vi "From Value.vi"(8 "error in (no error)":errorcluster, 10 "PV Data in":refnum<class "PV Data.lvclass">, 11 "NT Scalar (Numeric) in":refnum<class "NT Scalar (Numeric).lvclass">) -> (0 "error out":errorcluster, 2 "PV Data out":refnum<class "PV Data.lvclass">, 3 "NT Scalar (Numeric) out":refnum<class "NT Scalar (Numeric).lvclass">)   [LabVIEW 2020, in "PV Access.lvlib" / "PV Data.lvlib" / "NT Scalar (Numeric).lvclass"]
uses:
  NT Scalar (Numeric).lvclass
  NT Scalar (Numeric).lvclass/NT Scalar (Numeric).ctl
  PV Data/PV Data.lvclass
  NT Scalar/NT Scalar.lvclass
  PV Data/Read Field (String).vi
  PV Data/Read Field (Variant).vi
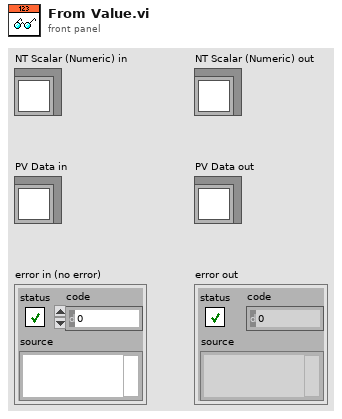
[diagram p1: front panel]
types:
  T1 = typedef "PV Access.lvlib/PV Data.lvlib/Alarm Limits.ctl" = cluster{"Active":bool, "Low Alarm Limit":variant, "Low Warning Limit":variant, "High Warning Limit":variant, "High Alarm Limit":variant, "Low Alarm Severity":T2, "Low Warning Severity":T2, "High Warning Severity ":T2, "High Alarm Severity":T2, "Hysteresis":dbl}
  T2 = typedef "PV Access.lvlib/PV Data.lvlib/Alarm Severity.ctl" = enum32{"no", "minor", "major", "record", "invalid", "undefined", ""}
  T3 = typedef "PV Access.lvlib/PV Data.lvlib/Control Metadata.ctl" = cluster{"Limit Low":variant, "Limit High":variant, "Min Step":variant}
  T4 = typedef "PV Access.lvlib/PV Data.lvlib/Display Form.ctl" = enum32{"Default", "String", "Binary", "Decimal", "Hex", "Exponential", "Engineering"}
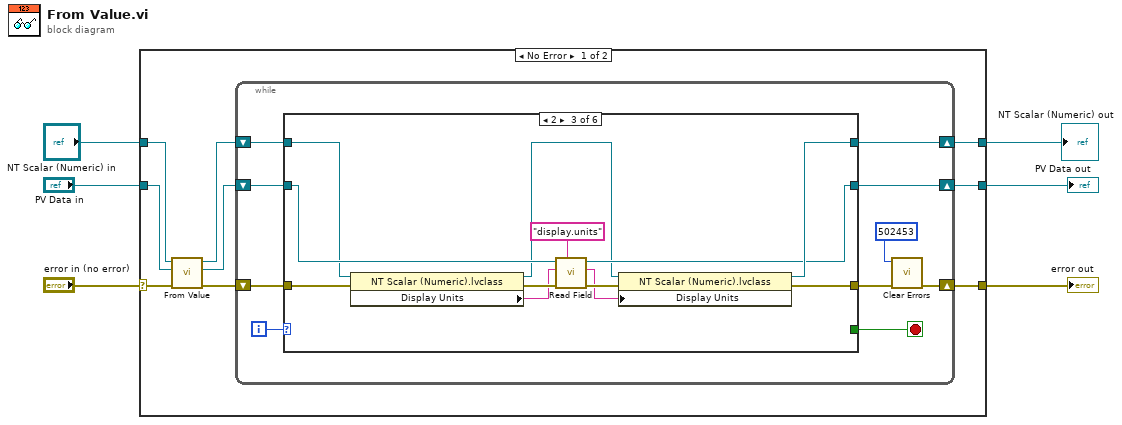
[diagram p0: block diagram]
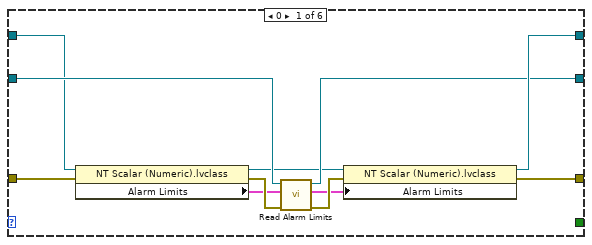
[diagram p2: hidden frame]
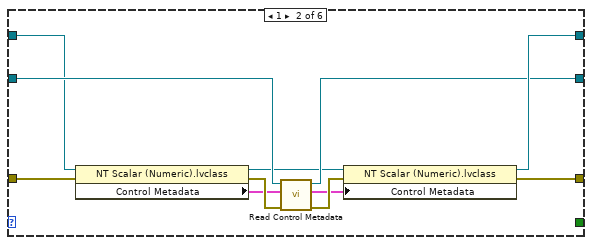
[diagram p3: hidden frame]
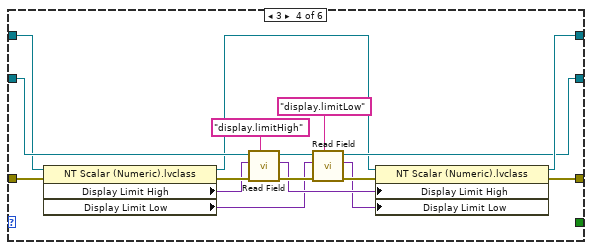
[diagram p4: hidden frame]
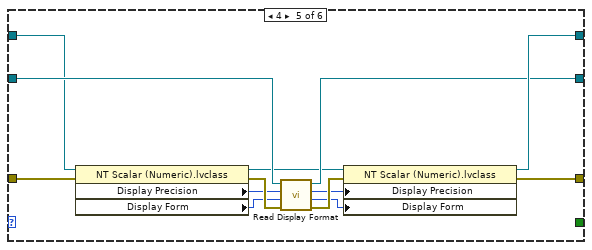
[diagram p5: hidden frame]
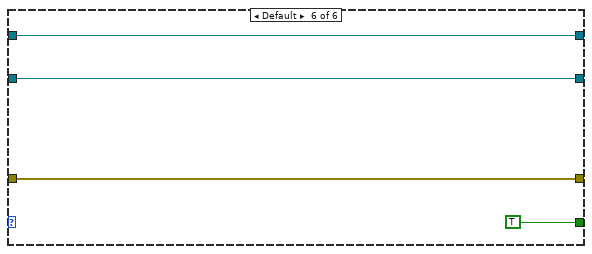
[diagram p6: hidden frame]
diagram:
  n1 = case shown="No Error" "error in (no error)" {
    selector: "error in (no error)" -> [w14 w96]
    tunnel: [w9 w96] -> w6
    tunnel: [w8 w94] -> w5
    tunnel: [w7 w95] -> w4
    tunnel: "PV Data in" -> [w13 w94]
    tunnel: "NT Scalar (Numeric) in" -> [w12 w95]
    frame No Error {
      n2 = call-parent "From Value.vi"("error in (no error)"=w14, "PV Data in"=w13, "NT Base in"=w12) -> ("error out"=w15:errorcluster, "PV Data out"=w11:refnum<class "PV Data.lvclass">, "NT Base out"=w10:refnum<class "NT Scalar (Numeric).lvclass">)  [unwired: 6 in]
      n3 = while {
        shift-right: [w21] -> w9
        shift-left: w15 -> [w23]
        shift-right: [w16] -> w8
        shift-left: w11 -> [w19]
        shift-right: [w17] -> w7
        shift-left: w10 -> [w18]
        i -> [w25]
        stop <- w24 stop-if-true
        n4 = case shown="2" w25 {
          tunnel: [_ _ _ _ _ TRUE] -> w24
          tunnel: w23 -> [w29 w40 w52 w67 w82 w92]
          tunnel: [w36 w47 w59 w76 w89 w92] -> w20
          tunnel: w19 -> [w34 w44 w53 w73 w87 w90]
          tunnel: w18 -> [w27 w38 w48 w61 w79 w91]
          tunnel: [w33 w43 w58 w75 w88 w91] -> w17
          tunnel: [w32 w42 w54 w69 w86 w90] -> w16
          frame 0 {
            n5 = property class="NT Scalar (Numeric).lvclass"(reference=w27, error in=w29) -> (reference out=w26:refnum<class "NT Scalar (Numeric).lvclass">, error out=w30:errorcluster, "Alarm Limits"=w28:T1)
            n6 = call "Read Alarm Limits.vi"("error in"=w30, "alarm limits in"=w28, "PV Data in"=w34) -> ("error out"=w35:errorcluster, "alarm limits out"=w31:T1, "PV Data out"=w32:refnum<class "PV Data.lvclass">)  [unwired: 5 in, 1 out]
            n7 = property class="NT Scalar (Numeric).lvclass"(reference=w26, error in=w35, "Alarm Limits"=w31) -> (reference out=w33:refnum<class "NT Scalar (Numeric).lvclass">, error out=w36:errorcluster)
          }
          frame 1 {
            n8 = property class="NT Scalar (Numeric).lvclass"(reference=w38, error in=w40) -> (reference out=w39:refnum<class "NT Scalar (Numeric).lvclass">, error out=w41:errorcluster, "Control Metadata"=w37:T3)
            n9 = call "Read Control Metadata.vi"("error in"=w41, "control metadata in"=w37, "PV Data in"=w44) -> ("error out"=w46:errorcluster, "control metadata out"=w45:T3, "PV Data out"=w42:refnum<class "PV Data.lvclass">)  [unwired: 5 in, 1 out]
            n10 = property class="NT Scalar (Numeric).lvclass"(reference=w39, error in=w46, "Control Metadata"=w45) -> (reference out=w43:refnum<class "NT Scalar (Numeric).lvclass">, error out=w47:errorcluster)
          }
          frame 2 {
            n11 = property class="NT Scalar (Numeric).lvclass"(reference=w48, error in=w52) -> (reference out=w49:refnum<class "NT Scalar (Numeric).lvclass">, error out=w51:errorcluster, "Display Units"=w50:string)
            n12 = call-poly "Read Field.vi"("field name"="display.units", "error in (no error)"=w51, "default"=w50, "PV Data in"=w53) -> ("error out"=w56:errorcluster, "value"=w55:string, "PV Data out"=w54:refnum<class "PV Data.lvclass">)  [unwired: 5 in]
            n13 = property class="NT Scalar (Numeric).lvclass"(reference=w49, error in=w56, "Display Units"=w55) -> (reference out=w58:refnum<class "NT Scalar (Numeric).lvclass">, error out=w59:errorcluster)
          }
          frame 3 {
            n14 = property class="NT Scalar (Numeric).lvclass"(reference=w61, error in=w67) -> (reference out=w60:refnum<class "NT Scalar (Numeric).lvclass">, error out=w66:errorcluster, "Display Limit High"=w65:variant, "Display Limit Low"=w63:variant)
            n15 = call-poly "Read Field.vi"("field name"="display.limitHigh", "error in (no error)"=w66, "value"=w65, "PV Data in"=w73) -> ("error out"=w72:errorcluster, "value out"=w64:variant, "PV Data out"=w70:refnum<class "PV Data.lvclass">)  [unwired: 4 in, 1 out]
            n16 = call-poly "Read Field.vi"("field name"="display.limitLow", "error in (no error)"=w72, "value"=w63, "PV Data in"=w70) -> ("error out"=w71:errorcluster, "value out"=w62:variant, "PV Data out"=w69:refnum<class "PV Data.lvclass">)  [unwired: 4 in, 1 out]
            n17 = property class="NT Scalar (Numeric).lvclass"(reference=w60, error in=w71, "Display Limit High"=w64, "Display Limit Low"=w62) -> (reference out=w75:refnum<class "NT Scalar (Numeric).lvclass">, error out=w76:errorcluster)
          }
          frame 4 {
            n18 = property class="NT Scalar (Numeric).lvclass"(reference=w79, error in=w82) -> (reference out=w80:refnum<class "NT Scalar (Numeric).lvclass">, error out=w81:errorcluster, "Display Precision"=w78:i32, "Display Form"=w77:T4)
            n19 = call "Read Display Format.vi"("error in"=w81, "form in"=w77, "precision in"=w78, "PV Data in"=w87) -> ("error out"=w85:errorcluster, "form"=w83:T4, "precision"=w84:i32, "PV Data out"=w86:refnum<class "PV Data.lvclass">)  [unwired: 4 in]
            n20 = property class="NT Scalar (Numeric).lvclass"(reference=w80, error in=w85, "Display Precision"=w84, "Display Form"=w83) -> (reference out=w88:refnum<class "NT Scalar (Numeric).lvclass">, error out=w89:errorcluster)
          }
          frame Default {
          }
        }
        n21 = call <vilib>:"Clear Errors.vi"("error in (no error)"=w20, "specific error code to clear (0: all)"=502453) -> ("error out"=w21:errorcluster)  [unwired: 4 in, 1 out]
      }
    }
    frame Error {
    }
  }
  "error out" <- w6
  "NT Scalar (Numeric) out" <- w4
  "PV Data out" <- w5
